vi "testing stimulator configuration_v2.vi"() -> ()   [LabVIEW 2021]
uses:
  type-defs/odor description array (type def).ctl
  type-defs/odor info cluster (type def).ctl
  type-defs/odor selection (type def).ctl
  type-defs/odor color (type def).ctl
  e7995511-3971-4f63-b655-b8bfcb8d6523.vi
panel:
  out "error out":errorcluster
  in  "error in (no error)":errorcluster
  in  "Stop":bool
  in  "Reset":bool
  in  "odor descriptions":T1
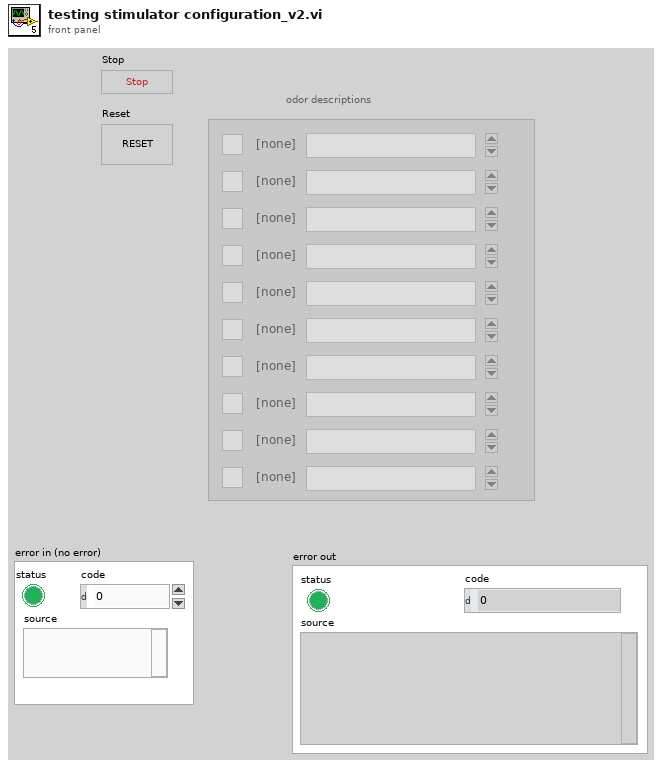
[diagram p1: front panel]
types:
  T1 = typedef "odor description array (type def).ctl" = T2[]
  T2 = typedef "odor info cluster (type def).ctl" = cluster{"odor channel":T3, "odor description":string, "odor color":T4, "odor channel active":bool}
  T3 = typedef "odor selection (type def).ctl" = enum16{"[none]", "odor 1", "odor 2", "odor 3", "odor 4", "odor 5", "odor 6", "odor 7", "odor 8", "odor 9", "odor 10"}
  T4 = typedef "odor color (type def).ctl" = u16
  T5 = enum8{"Enabled", "Disabled", "Disabled and Grayed Out"}
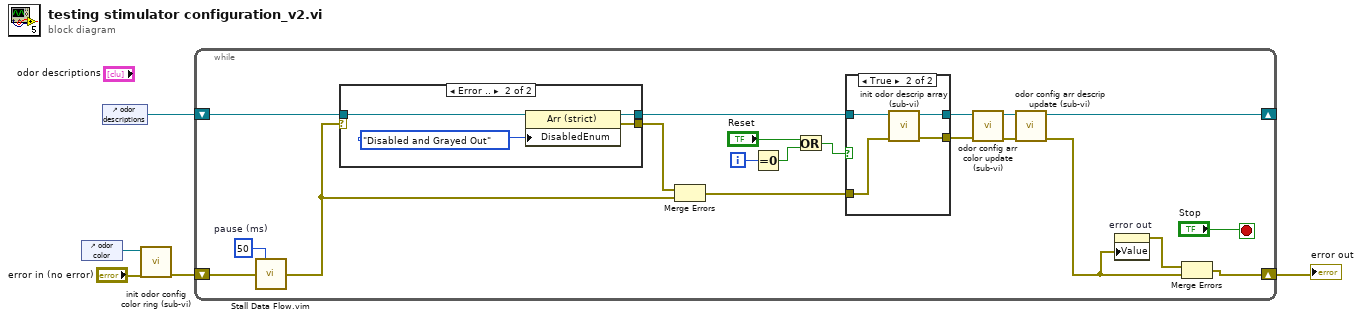
[diagram p0: block diagram]
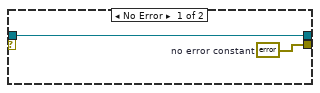
[diagram p2: hidden frame]
diagram:
  n1 = control-ref of="odor color"() -> (w4:refnum<vi>)
  n2 = control-ref of="odor descriptions"() -> (w5:refnum<vi>)
  n3 = call "init odor config color ring (sub-vi).vi"("error in (no error)"="error in (no error)", "ring refnum"=w4) -> ("error out"=w2:errorcluster)  [unwired: 8 in, 1 out]
  n4 = while {
    shift-right: [w19] -> w1
    shift-left: w2 -> [w8]
    shift-right: [w13] -> _
    shift-left: w5 -> [w12]
    i -> [w23]
    stop <- "Stop" stop-if-true
    w9 = u32 50  # pause (ms)
    n5 = call "Stall Data Flow.vim"("value in"=w8, "milliseconds to wait"=w9) -> ("value out"=w6:errorcluster)  [unwired: 1 out]
    n6 = case shown="Error .." w6 {
      tunnel: w12 -> [w27 w31]
      tunnel: [w27 w30] -> w11
      tunnel: [w26 w29] -> w10
      frame No Error {
        w26 = errorcluster {"status"=FALSE, "code"=0, "source"=""}  # no error constant
      }
      frame Error {
        n7 = property class="Arr (strict)"(reference=w31, "DisabledEnum"=T5."Disabled and Grayed Out" ("Disabled")) -> (reference out=w30:refnum<vi>, error out=w29:errorcluster)  [unwired: 1 in]
      }
    }
    n8 = Merge Errors(w10, w6) -> (w7:errorcluster)
    n9 = Equal To 0?(x=w23) -> (x = 0?=w22:bool)
    n10 = Or(x="Reset", y=w22) -> (x .or. y?=w25:bool)
    n11 = case shown="True" w25 {
      tunnel: w11 -> [w33 w37]
      tunnel: w7 -> [w32 w35]
      tunnel: [w32 w34] -> w17
      tunnel: [w33 w36] -> w18
      frame False {
      }
      frame True {
        n12 = call "init odor descrip array (sub-vi).vi"("error in (no error)"=w35, "array refnum"=w37) -> ("error out"=w34:errorcluster, "array refnum out"=w36:refnum<vi>)  [unwired: 8 in]
      }
    }
    n13 = call "odor config arr color update (sub-vi).vi"("error in (no error)"=w17, "array refnum"=w18) -> ("error out"=w15:errorcluster, "array refnum out"=w16:refnum<vi>)  [unwired: 8 in]
    n14 = call "odor config arr descrip update (sub-vi).vi"("error in (no error)"=w15, "array refnum"=w16) -> ("error out"=w14:errorcluster, "array refnum out"=w13:refnum<vi>)  [unwired: 8 in]
    n15 = property on="error out" class="Clust (strict)"("Value"=w14) -> (error out=w20:errorcluster)  [unwired: 2 in, 1 out]
    n16 = Merge Errors(w20, w14) -> (w19:errorcluster)
  }
  "error out" <- w1
